vi "sccx.vi"(0 "IP adress":string="192.109.209.229", 1 "stop":bool, 2 "Channel":u8(ring) items=["1", "2", "3", "4", "5", "6", "7", "8", "9", "10", "11", "12", "13", "14", "15", "16"], 4 "Exit":bool, 5 "Start":bool, 6 "Draw":enum16{"Ewe(t)", "Ece(t)", "I(t)", "Q(t)"}(ring)) -> (7 "XY Graph":cluster{"Data 101":sgl[], "Data 101":sgl[]}(graph), 8 "Number of points":i32=1992)   [LabVIEW 2014]
doc: "Chrono-Amperometry (CA) is a controlled-potential technique. The current response is measured to an applied potential step.\nIn general, in this VI, the first thing to do is to start by establishing the connection with the instrument defined by its IP adress, then load the firmware in the channel selected, get the information on the plugged channels, load protocol on a channel, start/stop the protocol, retreive data and draw the graph."
uses:
  LLB/dll_Functions.llb/SCCXParameters.ctl
panel:
  in  "Display Parameters?":bool caption="Display Parameters"
  out "DllPath":path caption="DLL Path"
  out "LibVersion":string caption="DLL Version"
  in  "SCCX Parameters":T1={"I_Range"=11, "E_Range"=0, "Bandwidth"=3, "par_E0"=1.0, "par_A"=0.0, "par_B"=0.1, "par_QRP_select"=1, "par_E_duration"=0.01, "par_E_dt_rec"=0.0001, "par_I0_duration"=0.01, "par_I0_dt_rec"=0.0001, "par_NC"=9, "par_RC"=1, "par_Q_limit_val"=5e-05, "par_Q_limit_cfg"=0, "par_QRP_time"=0.005, "ce"=0, "em"=0} {"par_Q_limit_cfg" items=["Disable"=0, "Enable if <"=129, "Enable if >"=133]; "par_QRP_select" items=["Ewe", "Ece"]; "E_Range" items=["±2.5V", "±5V", "±10V", "Auto"]; "Bandwidth" items=["1"=1, "2"=2, "3"=3, "4"=4, "5"=5, "6"=6, "7"=7, "8"=8, "9"=9]; "I_Range" items=["1pA", "1nA", "10nA", "100nA", "1µA", "10µA", "100µA", "1mA", "10mA", "100mA", "1A", "Booster", "Auto"]}
  out "Exit 2":bool=TRUE
  out "Data 174":sgl[][](array[numeric]) format="%.2f"
  # "Instructions:\nBefore running the VI you must type a valid IP adress that corresponds to the instrument.Then press the Run button to execute this VI.\nWhile this VI is running, choose the available channel, enter the CA parameters or keep the default values, then press the start button to begin the experience.\nChoose the waveform to draw (Ewe(t) or I(t)). You can stop the measure if you press the stop button and exit the execution if you press the exit button."
  # "V"
  # "Next En+1 = En - B * (A - QRP)"
  # "s"
  # "s"
  # "Switch to  I = 0"
  # "s"
  # "s"
  # "s"
  # "C"
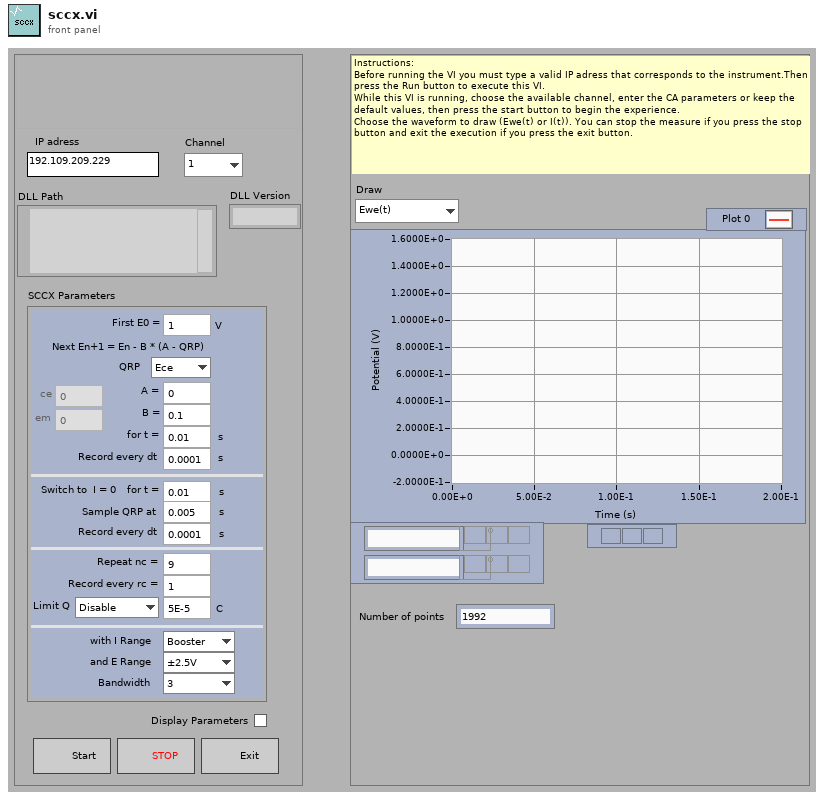
[diagram p1: front panel]
types:
  T1 = typedef "SCCXParameters.ctl" = cluster{"I_Range":u16, "E_Range":u16, "Bandwidth":u16, "par_E0":sgl, "par_A":sgl, "par_B":sgl, "par_QRP_select":u16, "par_E_duration":sgl, "par_E_dt_rec":sgl, "par_I0_duration":sgl, "par_I0_dt_rec":sgl, "par_NC":i32, "par_RC":i32, "par_Q_limit_val":sgl, "par_Q_limit_cfg":u16, "par_QRP_time":sgl, "ce":i32, "em":i32}
  T2 = cluster{"LibVersion":string, "StringLength":u32, "DllPath":path}
  T3 = cluster{"Channel":i32, "BoardVersion":i32, "BoardSerialCode":i32, "FirmwareCode":i32, "FirmwareVersion":i32, "XilinxVersion":i32, "AmpCode":i32, "NbAmp":i32, "LcBoard":i32, "Zboard":i32, "MuxBoard":i32, "GPRAboard":i32, "MemSize":i32, "MemFilled":i32, "state":i32, "MaxIRange":i32, "MinIRange":i32, "MaxBandwidth":i32, "NbOfTechniques":i32}
  T4 = typedef "TechniqueParameters.ctl" = cluster{"String Label":string, "Type":i32, "Valeur":i32, "Index":i32}
  T5 = cluster{"string before end tag":string, i32, i32, i32}[]
  T6 = cluster{"IRQskipped":i32, "NbRaws":i32, "NbCols":i32, "Technique Index":i32, "TechniqueID":i32, "PrcessIndex":i32, "loop":i32, "StartTime":dbl, "MuxPad":i32}
  T7 = cluster{"State":i32, "MemFilled":i32, "TimeBase":sgl, " Ewe":sgl, " EweRangeMin":sgl, " EweRangeMax":sgl, "Ece":sgl, "EceRangeMin":sgl, "EceRangeMax":sgl, "Eoverflow":i32, "I":sgl, "IRange":i32, "Ioverflow":i32, "ElapsedTime":sgl, "Freq":sgl, "Rcomp":sgl, "Saturation":sgl, "OptErr":i32, "OptPos":i32}
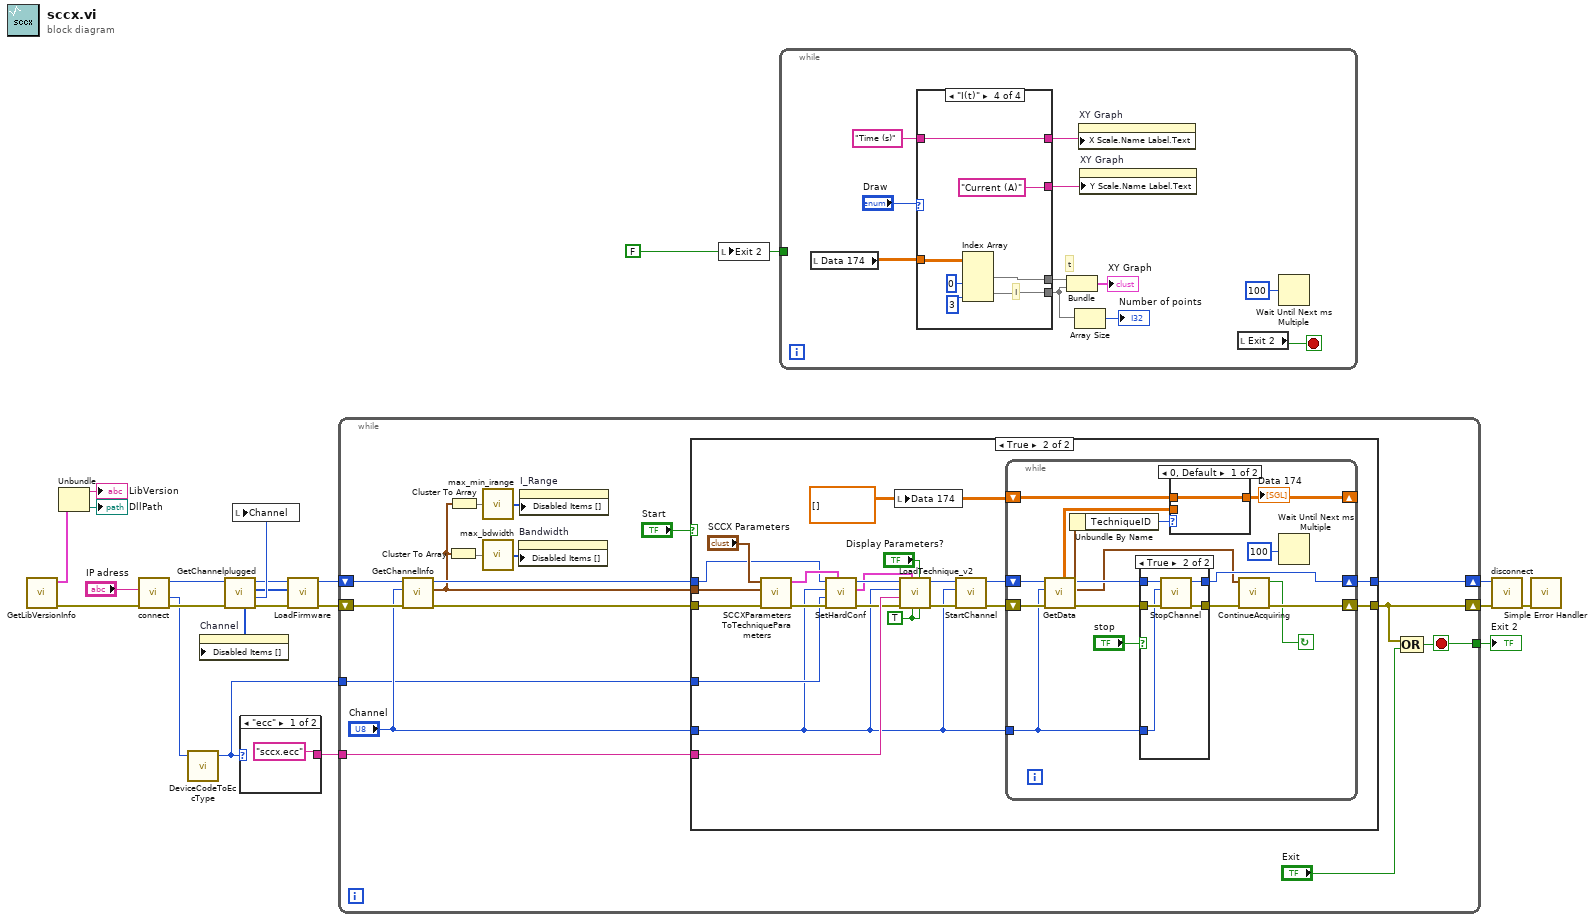
[diagram p0: block diagram]
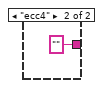
[diagram p2: hidden frame]
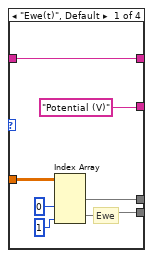
[diagram p3: hidden frame]
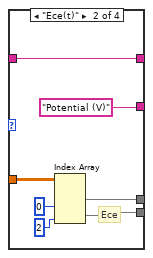
[diagram p4: hidden frame]
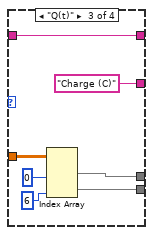
[diagram p5: hidden frame]
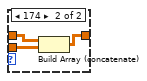
[diagram p8: hidden frame]
diagram:
  w21 = FALSE ("Exit 2")
  n1 = call "GetLibVersionInfo.vi"() -> ("error out"=w1:errorcluster, "LibInfo"=w4:T2)  [unwired: 10 in]
  n2 = Unbundle(w4) -> ("LibVersion"=→"LibVersion":string, "DllPath"=→"DllPath":path)  [unwired: 1 out]
  n3 = call "connect.vi"("error in (no error)"=w1, "IP"="IP adress") -> ("error out"=w18:errorcluster, "Device Code"=w8:i32, "ID Out"=w13:i32)  [unwired: 6 in, 1 out]
  n4 = call "DeviceCodeToEccType.vi"("Device Code"=w8) -> ("EccType"=w5:enum16{"ecc", "ecc4"})  [unwired: 4 in]
  n5 = call "GetChannelplugged.vi"("error in (no error)"=w18, "ID In"=w13) -> ("error out"=w15:errorcluster, "FirstPluggedChannel"=w19:u8, "PluggedChannels"=w9:u8[], "ID Out"=w14:i32, "DisabledChannels"=w17:i32[])  [unwired: 5 in]
  n6 = property on="Channel" class="Ring (strict)"("Disabled Items []"=w17) -> ()  [unwired: 2 in, 2 out]
  n7 = local write "Channel"(w19) -> ()
  n8 = case shown="\"ecc\"" w5 {
    tunnel: ["sccx.ecc" ("FName") "" ("FName")] -> w6
    frame "ecc" {
    }
    frame "ecc4" {
    }
  }
  n9 = call "LoadFirmware.vi"("error in (no error)"=w15, "Channels"=w9, "ID In"=w14) -> ("error out"=w16:errorcluster, "ID Out"=w12:i32)  [unwired: 6 in, 1 out]
  n10 = while {
    shift-right: [w29] -> w11
    shift-left: w16 -> [w36]
    tunnel: [w27] -> w22
    shift-right: [w31] -> w10
    shift-left: w12 -> [w33]
    tunnel: w6 -> [w26]
    tunnel: w5 -> [w25]
    stop <- w27 stop-if-true
    n11 = call "GetChannelInfo.vi"("error in (no error)"=w36, "Channel"="Channel", "ID"=w33) -> ("error out"=w35:errorcluster, "Channel information"=w30:T3, "ID Out"=w32:i32)  [unwired: 6 in]
    n12 = Cluster To Array(cluster=w30) -> (array=w39:i32[])
    n13 = Cluster To Array(cluster=w30) -> (array=w40:i32[])
    n14 = call "max_min_irange.vi"("resources"=w40) -> ("disabled ranges"=w37:i32[])
    n15 = call "max_bdwidth.vi"("resources"=w39) -> ("disabled ranges"=w38:i32[])
    n16 = property on="Bandwidth" class="Ring (strict)"("Disabled Items []"=w38) -> ()  [unwired: 2 in, 2 out]
    n17 = property on="I_Range" class="Ring (strict)"("Disabled Items []"=w37) -> ()  [unwired: 2 in, 2 out]
    n18 = case shown="True" "Start" {
      tunnel: "Channel" -> [_ w45]
      tunnel: [w43 w64] -> w29
      tunnel: w35 -> [w43 w59]
      tunnel: w32 -> [w42 w47]
      tunnel: [w42 w54] -> w31
      tunnel: w30 -> [_ w60]
      tunnel: w26 -> [_ w53]
      tunnel: w25 -> [_ w46]
      frame False {
      }
      frame True {
        w58 = TRUE ("First Protocol")
        w63 = sgl[][] []
        n19 = call "SCCXParametersToTechniqueParameters.vi"("error in (no error)"=w59, "Channel information"=w60, "SCCX Parameters"="SCCX Parameters") -> ("error out"=w52:errorcluster, "TechniqueParameters"=w48:T4[])  [unwired: 7 in]
        n20 = call "SetHardConf.vi"("Params Values"=w48, "error in (no error)"=w52, "EccType"=w46, "Channel"=w45, "ID In"=w47) -> ("error out"=w51:errorcluster, "Params Values Trimed"=w49:T5, "ID Out"=w50:i32)  [unwired: 4 in]
        n21 = local write "Data 174"(w63) -> ()
        n22 = call "LoadTechnique_v2.vi"("Last Protocol"=w58, "Display Parameters?"="Display Parameters?", "First Protocol"=w58, "TechniqueParameters"=w49, "error in (no error)"=w51, "FName"=w53, "Selected Channel"=w45, "ID In"=w50) -> ("error out"=w57:errorcluster, "ID  Out"=w56:i32)  [unwired: 2 in]
        n23 = call "StartChannel.vi"("error in (no error)"=w57, "Channel"=w45, "ID In"=w56) -> ("error out"=w61:errorcluster, "ID Out"=w55:i32)  [unwired: 7 in]
        n24 = while {
          shift-right: [w69] -> w64
          shift-left: w61 -> [w81]
          shift-right: [w78] -> _
          shift-left: w63 -> [w79]
          shift-right: [w70] -> w54
          shift-left: w55 -> [w72]
          tunnel: w45 -> [w65]
          stop <- w66 continue-if-true
          n25 = call "GetData.vi"("error in (no error)"=w81, "Channel"=w65, "ID In"=w72) -> ("error out"=w77:errorcluster, "Data information"=w75:T6, "Current values"=w67:T7, "ID Out"=w71:i32, "Data"=w73:dbl[][])  [unwired: 4 in]
          n26 = Unbundle By Name(w75) -> ("TechniqueID"=w74:i32)
          n27 = case shown="True" "stop" {
            tunnel: [w83 w88] -> w68
            tunnel: w77 -> [w83 w87]
            tunnel: w71 -> [w82 w86]
            tunnel: [w82 w85] -> w70
            tunnel: w65 -> [_ w84]
            frame False {
            }
            frame True {
              n28 = call "StopChannel.vi"("error in (no error)"=w87, "Channel"=w84, "ID In"=w86) -> ("error out"=w88:errorcluster, "ID Out"=w85:i32)  [unwired: 7 in]
            }
          }
          n29 = case shown="0, Default" w74 {
            tunnel: w73 -> [_ w92]
            tunnel: w79 -> [w89 w91]
            tunnel: [w89 w90] -> w78
            frame 0, Default {
            }
            frame 174 {
              n30 = Build Array (concatenate)(w91, w92) -> (w90:dbl[][])
            }
          }
          "Data 174" <- w78
          n31 = call "ContinueAcquiring.vi"("error in"=w68, "Current values"=w67) -> ("error out"=w69:errorcluster, "ContinueAcquiring?"=w66:bool)  [unwired: 8 in]
          n32 = Wait Until Next ms Multiple(millisecond multiple=u32 100) -> ()  [unwired: 1 out]
        }
      }
    }
    n33 = Compound Arithmetic op=OR(w29, "Exit") -> (w27:bool)
  }
  "Exit 2" <- w22
  n34 = local write "Exit 2"(w21) -> ()
  n35 = while {
    tunnel: w21 -> [_]
    stop <- w102 stop-if-true
    # "t"
    n36 = local read "Data 174"() -> (w97:sgl[][])
    n37 = case shown="\"I(t)\"" "Draw" {
      tunnel: ["Potential (V)" ("Y Scale.Name Label.Text") "Potential (V)" ("Y Scale.Name Label.Text") "Charge (C)" ("Y Scale.Name Label.Text") "Current (A)" ("Y Scale.Name Label.Text")] -> w100
      tunnel: [w110 w117 w124 w131] -> w99
      tunnel: "Time (s)" ("Y Scale.Name Label.Text") -> [w110 w117 w124 w131]
      tunnel: w97 -> [w107 w114 w122 w128]
      tunnel: [w105 w112 w119 w126] -> w95
      tunnel: [w104 w111 w118 w125] -> w94
      frame "Ewe(t)", Default {
        # "Ewe"
        n38 = Index Array(array=w107, index (col) #1=0 ("Index"), index (col) #2=1 ("Index")) -> (element #1=w105:sgl[], element #2=w104:sgl[])  [unwired: 2 in]
      }
      frame "Ece(t)" {
        # "Ece"
        n39 = Index Array(array=w114, index (col) #1=0 ("Index"), index (col) #2=2 ("Index")) -> (element #1=w112:sgl[], element #2=w111:sgl[])  [unwired: 2 in]
      }
      frame "Q(t)" {
        n40 = Index Array(array=w122, index (col) #1=0 ("Index"), index (col) #2=6 ("indice désactivé (col)")) -> (element #1=w119:sgl[], element #2=w118:sgl[])  [unwired: 2 in]
      }
      frame "I(t)" {
        # "I"
        n41 = Index Array(array=w128, index (col) #1=0 ("Index"), index (col) #2=3 ("indice désactivé (col)")) -> (element #1=w126:sgl[], element #2=w125:sgl[])  [unwired: 2 in]
      }
    }
    n42 = Bundle("Data 174"=w95, "Data 174"=w94) -> (→"XY Graph":cluster{"Data 174":sgl[], "Data 174":sgl[]})  [unwired: 1 in]
    n43 = Array Size(array=w94) -> (size(s)=→"Number of points":i32)
    n44 = property on="XY Graph" class="XYGraph (strict)"("X Scale.Name Label.Text"=w99) -> ()  [unwired: 2 in, 2 out]
    n45 = property on="XY Graph" class="XYGraph (strict)"("Y Scale.Name Label.Text"=w100) -> ()  [unwired: 2 in, 2 out]
    n46 = local read "Exit 2"() -> (w102:bool)
    n47 = Wait Until Next ms Multiple(millisecond multiple=u32 100) -> ()  [unwired: 1 out]
  }
  n48 = call "disconnect.vi"("error in (no error)"=w11, "ID In"=w10) -> ("error out"=w7:errorcluster)  [unwired: 9 in]
  n49 = call <vilib>:"Simple Error Handler.vi"("error in (no error)"=w7) -> ()  [unwired: 4 in, 5 out]
